vi "Main_v1.vi"() -> ()   [LabVIEW 2018, in "Application.lvlib"]
doc: "This VI is the main application VI in the Delacor QMH project template. This application VI is implemented as a simple state machine, which communicates with two different Delacor QMH modules.\n_____\nBased on DQMH Project Template 6.0.0.91."
uses:
  Application.lvlib
  Application Data--cluster.ctl
  Switches Module/MB switches Module.lvlib
  CE14 eMIC module/CE14 eMIC module.lvlib
  App States.ctl
  MB 01 switches Module/MB 01 switches Module.lvlib
  DMM Module/DMM Module.lvlib
  CE14  Module/CE14  Module.lvlib
  DRV cluster.ctl
  type defs/HW config.ctl
  Instrument Drivers/LVdriver_CE14(eMIC)/type defs/CE14.data.ctl
  Instrument Drivers/LVdriver_CE14(eMIC)/CE14_eMIC.lvlib
panel:
  out "eMIC response":T1[](array[typedef])
  out "time string":string
  out "Module ID":i32
  in  "Read ACI, ACV  from  eMIC(x6)":bool
  out "DCI":dbl
  out "DCV":dbl
  in  "Sets to Display":u16(ring)=2 items=["1st Display", "2nd Display", "1st & 2nd Display"]
  in  "Read DCI, DCV  from DMM":bool
  in  "Detector Rate":u8(ring)=2 items=["SLOW", "MID", "FAST"]
  in  "DCI range":dbl=10.0
  in  "DCV range":dbl=1000.0
  in  "config DMM":bool
  in  "mux2-1(DMM I) encode":enum16{"DMM I (0.5)", "DMM I (12)"}(ring)
  in  "DMM input Selection":bool
  in  "mux6_1(3wires)_encode":T2(ring)
  in  "mux6-1(x1)":bool
  in  "Time duration(ms)":i32
  in  "mux10_1(x6)_encode":T3(ring)
  in  "mux10-1(x6)":bool
  in  "eMIC (x6)":bool[](array[boolean])=[FALSE, FALSE, FALSE, FALSE, FALSE, FALSE]
  in  "eMIC":bool
  in  "demux1_10(x6)":T4(ring)
  in  "demux1-10(x6)":bool
  in  "SC enable":bool=TRUE
  in  "SC Enable":bool
  in  "M054 Close":bool
  in  "Arduino Close":bool
  in  "DMM Close":bool
  in  "M054 name":refnum<visa-resource-name>="COM11"
  in  "Arduino name":refnum<visa-resource-name>="COM16"
  in  "DMM name":refnum<visa-resource-name>="COM15"
  in  "M054 connect":bool
  in  "Arduino connect":bool
  in  "DMM connect":bool
  in  "Test":bool caption="Again"
  out "DMM Module Running?":bool
  out "MB01 Module Running?":bool
  in  "Start DMM Module Module":bool
  in  "Start MB01 Module Module":bool
  out "DRV 61":u32(colorbox)
  in  "Exit":bool
  in  "Pause":bool
  in  "Again":bool
  out "DRV 60":u32(colorbox) caption="60"
  out "DRV 59":u32(colorbox) caption="59"
  out "DRV 58":u32(colorbox) caption="58"
  out "DRV 57":u32(colorbox) caption="57"
  out "DRV 56":u32(colorbox) caption="56"
  out "DRV 55":u32(colorbox) caption="55"
  out "DRV 54":u32(colorbox) caption="54"
  out "DRV 53":u32(colorbox) caption="53"
  out "DRV 52":u32(colorbox) caption="52"
  out "DRV 51":u32(colorbox) caption="51"
  out "DRV 50":u32(colorbox) caption="50"
  out "DRV 49":u32(colorbox) caption="49"
  out "DRV 48":u32(colorbox) caption="48"
  out "DRV 47":u32(colorbox) caption="47"
  out "DRV 46":u32(colorbox) caption="46"
  out "DRV 45":u32(colorbox) caption="45"
  out "DRV 44":u32(colorbox) caption="44"
  out "DRV 43":u32(colorbox) caption="43"
  out "DRV 42":u32(colorbox) caption="42"
  out "DRV 41":u32(colorbox) caption="41"
  out "DRV 40":u32(colorbox) caption="40"
  out "DRV 39":u32(colorbox) caption="39"
  out "DRV 38":u32(colorbox) caption="38"
  out "DRV 37":u32(colorbox) caption="37"
  out "DRV 36":u32(colorbox) caption="36"
  out "DRV 35":u32(colorbox) caption="35"
  out "DRV 34":u32(colorbox) caption="34"
  out "DRV 33":u32(colorbox) caption="33"
  out "DRV 32":u32(colorbox) caption="32"
  out "DRV 31":u32(colorbox) caption="31"
  out "DRV 30":u32(colorbox) caption="30"
  out "DRV 29":u32(colorbox) caption="29"
  out "DRV 28":u32(colorbox) caption="28"
  out "DRV 27":u32(colorbox) caption="27"
  out "DRV 26":u32(colorbox) caption="26"
  out "DRV 25":u32(colorbox) caption="25"
  out "DRV 24":u32(colorbox) caption="24"
  out "DRV 23":u32(colorbox) caption="23"
  out "DRV 22":u32(colorbox) caption="22"
  out "DRV 21":u32(colorbox) caption="21"
  out "DRV 20":u32(colorbox) caption="20"
  out "DRV 19":u32(colorbox)=4375612 caption="19"
  out "DRV 18":u32(colorbox) caption="18"
  out "DRV 17":u32(colorbox) caption="17"
  out "DRV 16":u32(colorbox) caption="16"
  out "DRV 15":u32(colorbox) caption="15"
  out "DRV 14":u32(colorbox) caption="14"
  out "DRV 13":u32(colorbox)=4375612 caption="13"
  out "DRV 12":u32(colorbox) caption="12"
  out "DRV 11":u32(colorbox) caption="11"
  out "DRV 10":u32(colorbox) caption="10"
  out "DRV 9":u32(colorbox) caption="9"
  out "DRV 8":u32(colorbox) caption="8"
  out "DRV 7":u32(colorbox)=4375612 caption="7"
  out "DRV 6":u32(colorbox) caption="6"
  out "DRV 5":u32(colorbox) caption="5"
  out "DRV 4":u32(colorbox) caption="4"
  out "DRV 3":u32(colorbox) caption="3"
  out "DRV 2":u32(colorbox) caption="2"
  out "DRV 1":u32(colorbox)=13224393 caption="1"
  out "version":string caption="Version"
  in  "Hide Switches Module Module":bool
  in  "Show Switches Module Module":bool
  in  "Hide CE14 eMIC module Module":bool
  in  "Show CE14 eMIC module Module":bool
  in  "Stop CE14 eMIC module Module":bool
  in  "Stop Switches Module Module":bool
  in  "Start Switches Module Module":bool
  out "Active CE14 eMIC module Modules":string[](array[string])
  in  "Start New Instance CE14 eMIC module Module":bool
  in  "Select CE14 eMIC module Module Instance":i32(ring)=-1 items=["All"=-1]
  in  "Switches Module Module: Do Something Else":dbl caption="Do Something Else"
  in  "Switches Module Module: Do Something":bool
  out "Switches Module Running?":bool
  out "Status":string
  # "HV-60D: LED POWER DRIVER ON-LINE TESTER"
  # "DCI range:  10mV; 100mV;  1A, 10A"
  # "DCV range: 100mV/1V; 10V, 1000V"
  # "This top-level application allows you to launch and control a singleton module, and multiple instances of a cloneable module."
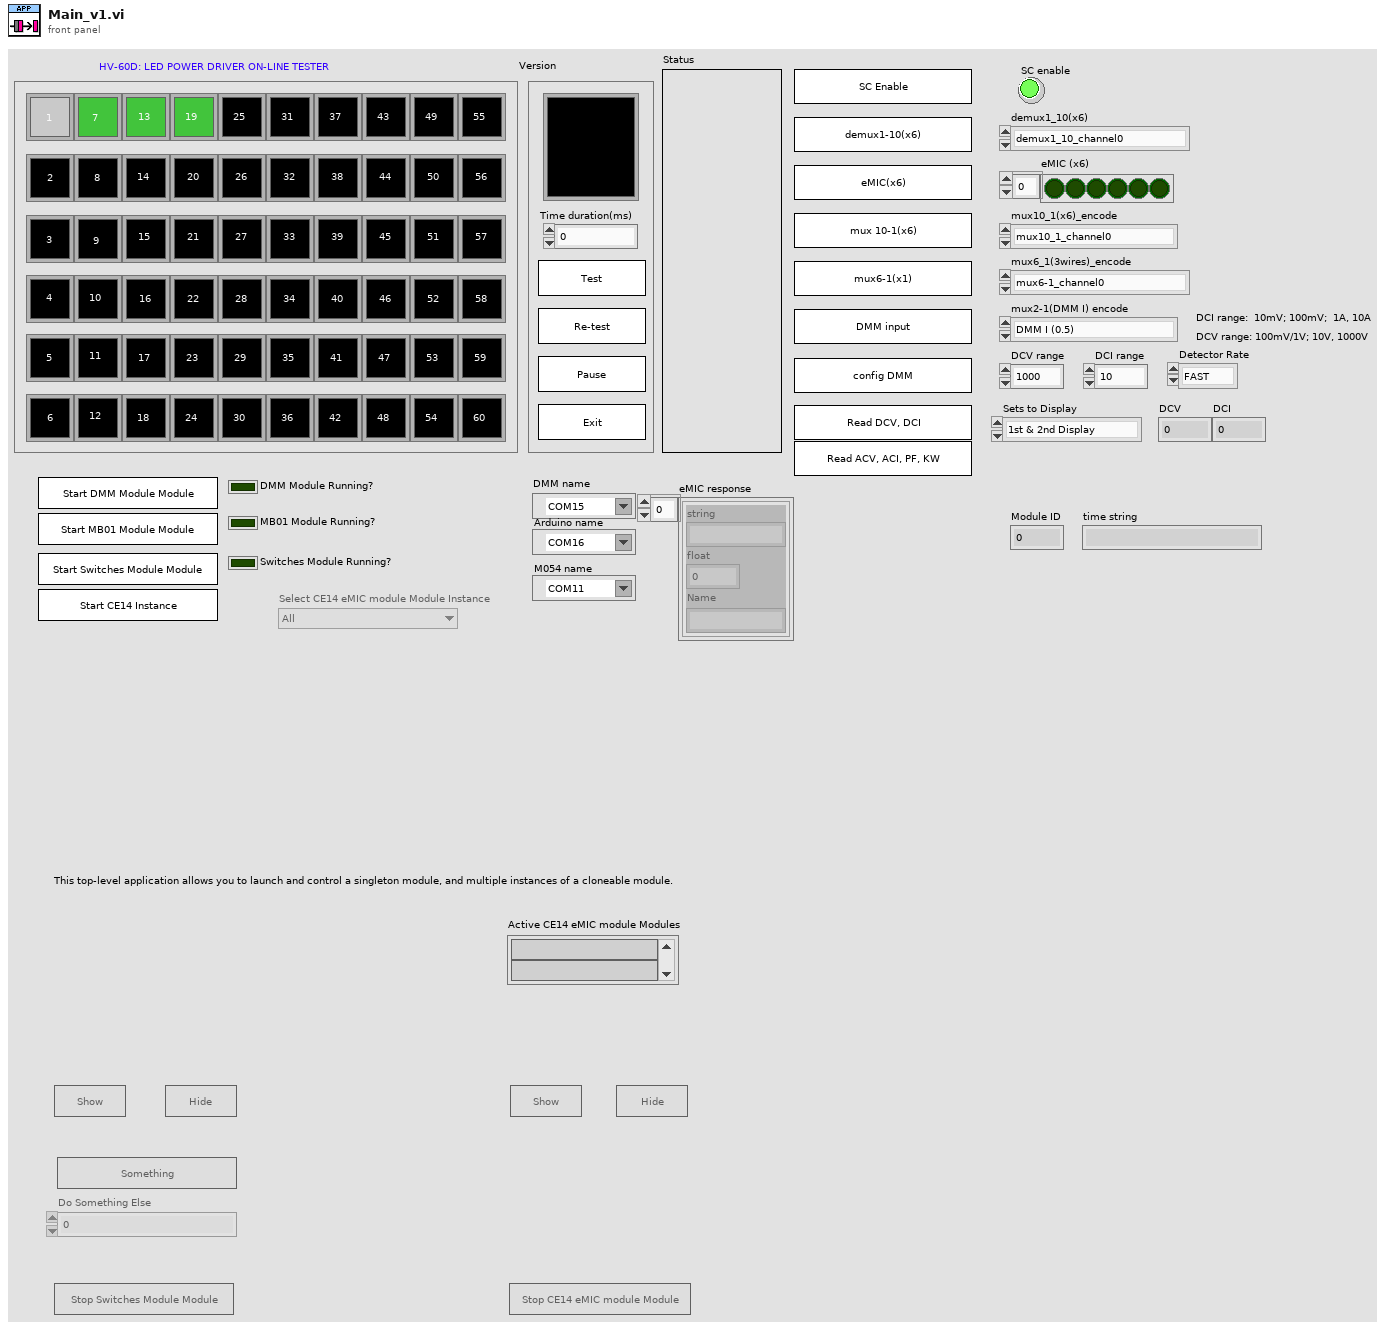
[diagram p1: front panel]
types:
  T1 = typedef "CE14_eMIC.lvlib/CE14.data.ctl" = cluster{"string":string, "float":dbl, "Name":string}
  T2 = enum16{"mux6-1_channel0", "mux6_1_channel1_0", "mux6_1_channel1_1", "mux6-1_channel1_2", "mux6_1_channel1_3", "mux6_1_channel2_0", "mux6_1_channel2_1", "mux6_1_channel2_2", "mux6_1_channel2_3", "mux6_1_channel3_0", "mux6_1_channel3_1", "mux6_1_channel3_2", "mux6_1_channel3_3", "mux6_1_channel4_0", "mux6_1_channel4_1", "mux6_1_channel4_2", "mux6_1_channel4_3", "mux6_1_channel5_0", "mux6_1_channel5_1", "mux6_1_channel5_2", "mux6_1_channel5_3", "mux6_1_channel6_0", "mux6_1_channel6_1", "mux6_1_channel6_2", "mux6_1_channel6_3"}
  T3 = enum16{"mux10_1_channel0", "mux10_1_channel1", "mux10_1_channel2", "mux10_1_channel3", "mux10_1_channel4", "mux10_1_channel5", "mux10_1_channel6", "mux10_1_channel7", "mux10_1_channel8", "mux10_1_channel9", "mux10_1_channel10"}
  T4 = enum16{"demux1_10_channel0", "demux1_10_channel1", "demux1_10_channel2", "demux1_10_channel3", "demux1_10_channel4", "demux1_10_channel5", "demux1_10_channel6", "demux1_10_channel7", "demux1_10_channel8", "demux1_10_channel9", "demux1_10_channel10"}
  T5 = typedef "Application.lvlib/App States.ctl" = enum16{"Apps.Initialize0", "Apps.Initialize1", "Apps.Initialize2", "Apps.Initialize3", "Apps.Initialize4", "Apps.Initialize Panel", "Apps.UI Interlocks", "Apps.UI.Reinitiatize", "Apps.Update Status", "Apps.Wait for Event", "Apps.Exit"}
  T6 = typedef "Application.lvlib/Application Data--cluster.ctl" = cluster{"Status":string, "Singleton Controls":refnum<vi>[], "Cloneable Controls":refnum<vi>[], "Module Ring Value":i32, "HW config":T7, "DUT values":T8[]}
  T7 = typedef "Application.lvlib/HW config.ctl" = cluster{"DMM":string, "mux":string, "demux":string, "eMIC1":string, "eMIC2":string, "eMIC3":string, "eMIC4":string, "eMIC5":string, "eMIC6":string}
  T8 = typedef "Application.lvlib/DRV cluster.ctl" = cluster{"Pass/Fail?":bool, "AC Characteristic":cluster{"Pass/Fail?":bool, "Voltage":cluster{"pass/fail?":bool, "Measured Value":dbl, "Upper Level":dbl, "Lower Level":dbl}, "Current":cluster{"pass/fail?":bool, "Measured Value":dbl, "Upper Level":dbl, "Lower Level":dbl}, "Power factor":cluster{"pass/fail?":bool, "Measured Value":dbl, "Upper Level":dbl, "Lower Level":dbl}, "Shorted Circuit":cluster{"Pass/Fail?":bool}}, "DC Characteristic":cluster{"Pass/Fail?":bool, "Voltage":cluster{"pass/fail?":bool, "Measured Value":dbl, "Upper Level":dbl, "Lower Level":dbl}, "Current":cluster{"pass/fail?":bool, "Measured Value":dbl, "Upper Level":dbl, "Lower Level":dbl}}}
  T9 = typedef "CE14  Module.lvlib/Broadcast Events--cluster.ctl" = cluster{"Module Did Init":refnum<user-event>, "Status Updated":refnum<user-event>, "Error Reported":refnum<user-event>, "Module Did Stop":refnum<user-event>, "Update Module Execution Status":refnum<user-event>, "eMICs response":refnum<user-event>}
  T10 = typedef "MB switches Module.lvlib/Broadcast Events--cluster.ctl" = cluster{"Module Did Init":refnum<user-event>, "Status Updated":refnum<user-event>, "Error Reported":refnum<user-event>, "Module Did Stop":refnum<user-event>, "Update Module Execution Status":refnum<user-event>}
  T11 = typedef "MB 01 switches Module.lvlib/Broadcast Events--cluster.ctl" = cluster{"Module Did Init":refnum<user-event>, "Status Updated":refnum<user-event>, "Error Reported":refnum<user-event>, "Module Did Stop":refnum<user-event>, "Update Module Execution Status":refnum<user-event>}
  T12 = typedef "DMM Module.lvlib/Broadcast Events--cluster.ctl" = cluster{"Module Did Init":refnum<user-event>, "Status Updated":refnum<user-event>, "Error Reported":refnum<user-event>, "Module Did Stop":refnum<user-event>, "Update Module Execution Status":refnum<user-event>}
  T13 = typedef "Application.lvlib/App States.ctl" = enum16{"Initialize", "Initialize Panel", "UI Interlocks", "Update Status", "Wait for Event", "Exit"}
  T14 = enum8{"Enabled", "Disabled", "Disabled and Grayed Out"}
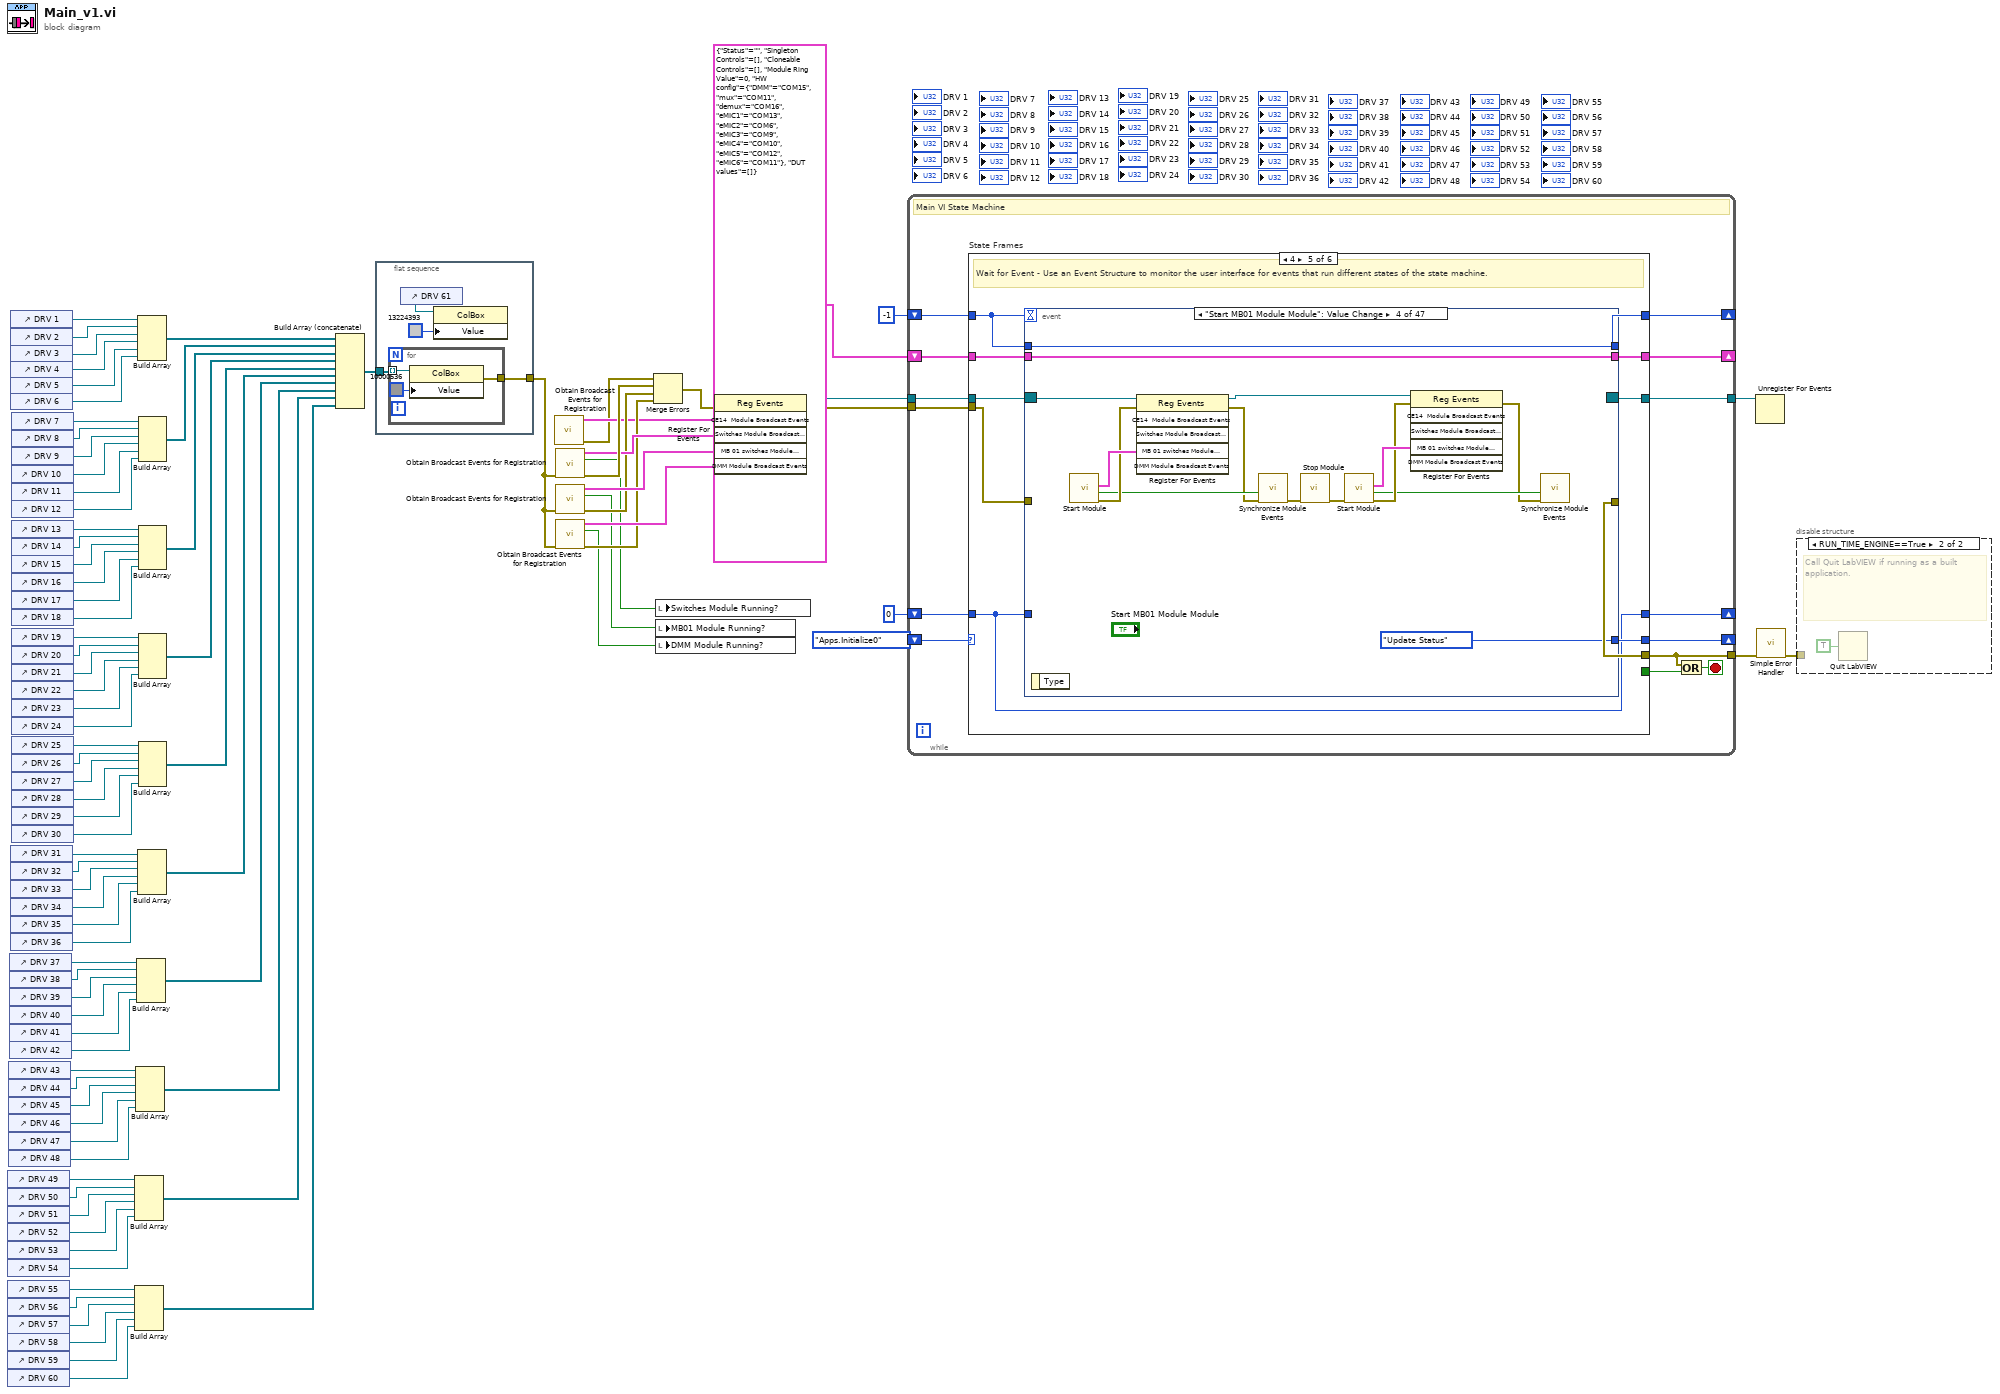
[diagram p0: block diagram]
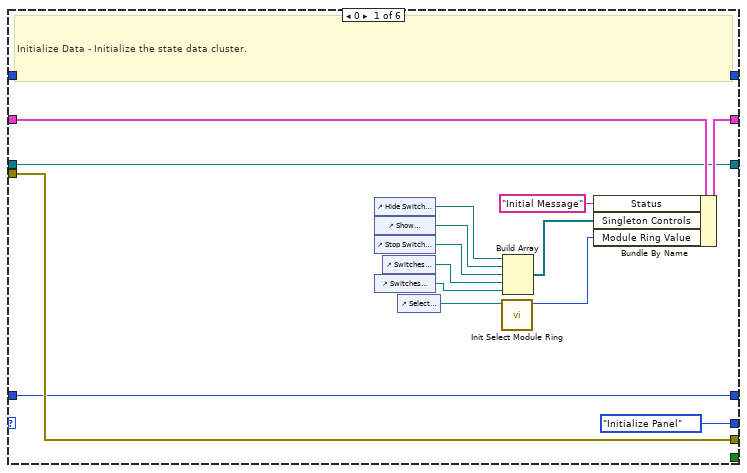
[diagram p2: hidden frame]
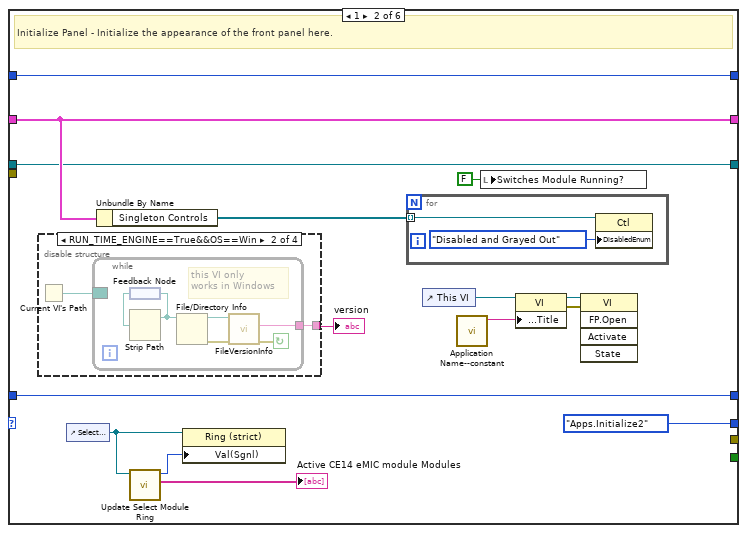
[diagram p3: hidden frame]
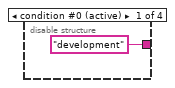
[diagram p4: hidden frame]
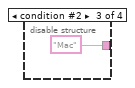
[diagram p5: hidden frame]
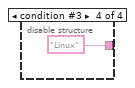
[diagram p6: hidden frame]
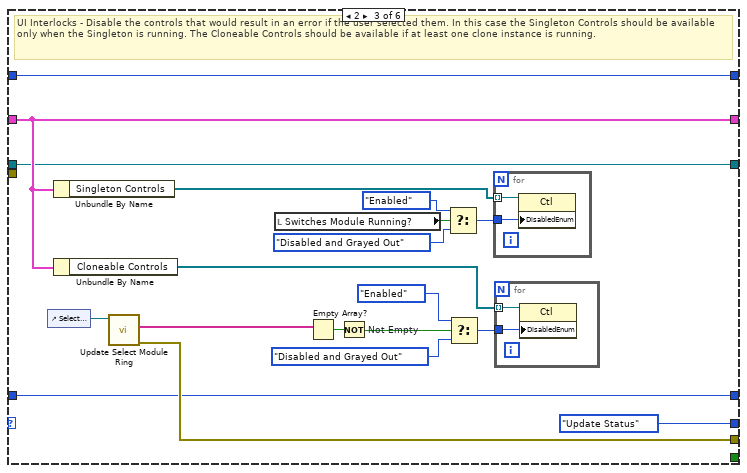
[diagram p7: hidden frame]
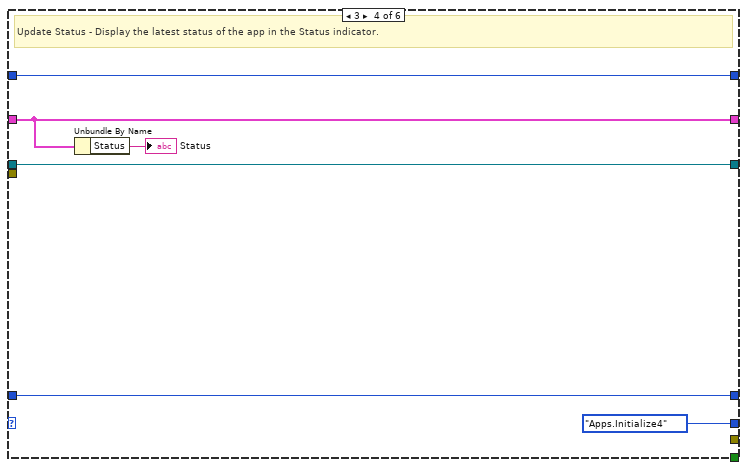
[diagram p8: hidden frame]
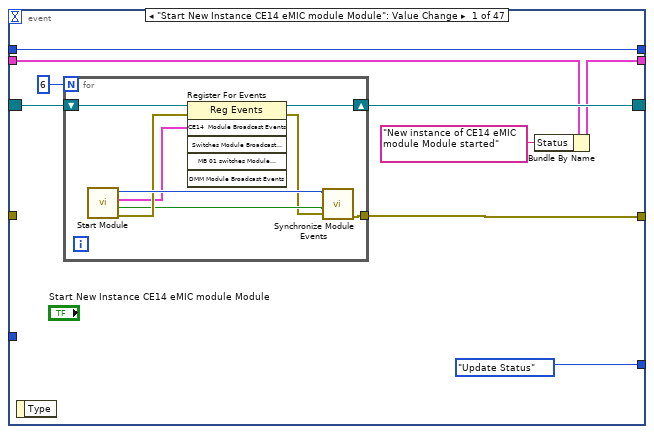
[diagram p9: hidden frame]
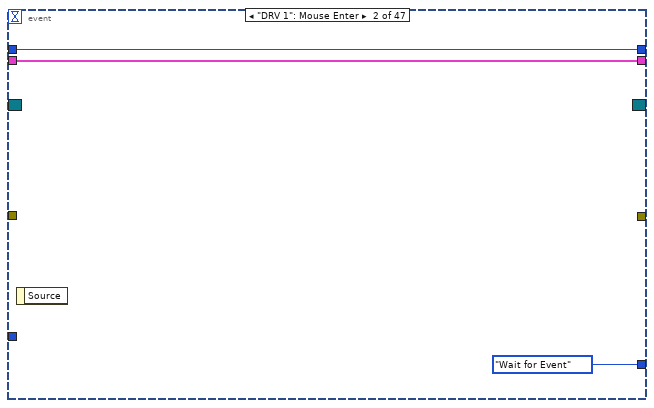
[diagram p10: hidden frame]
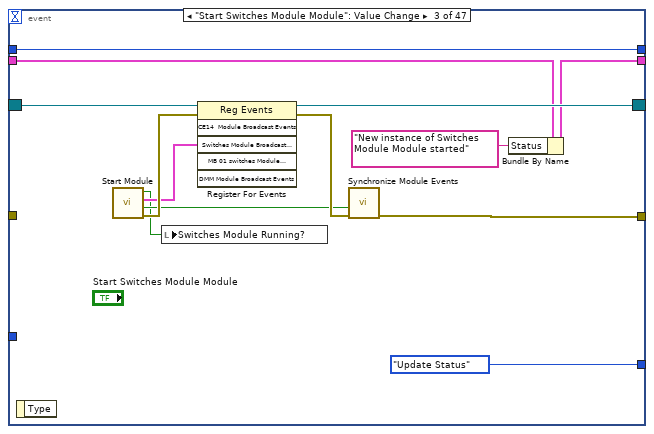
[diagram p11: hidden frame]
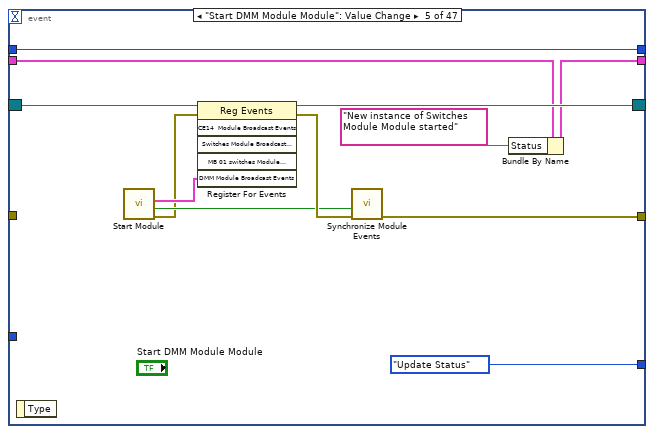
[diagram p12: hidden frame]
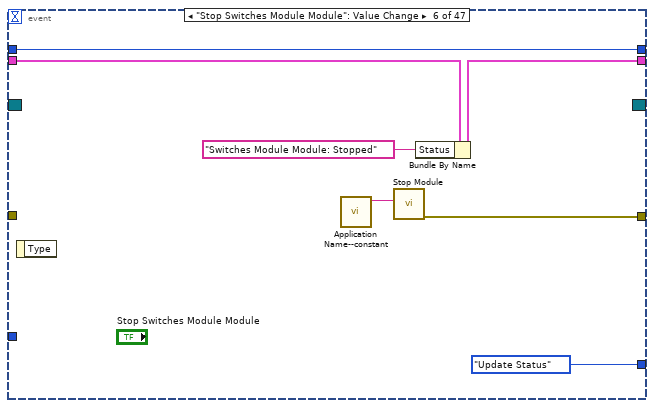
[diagram p13: hidden frame]
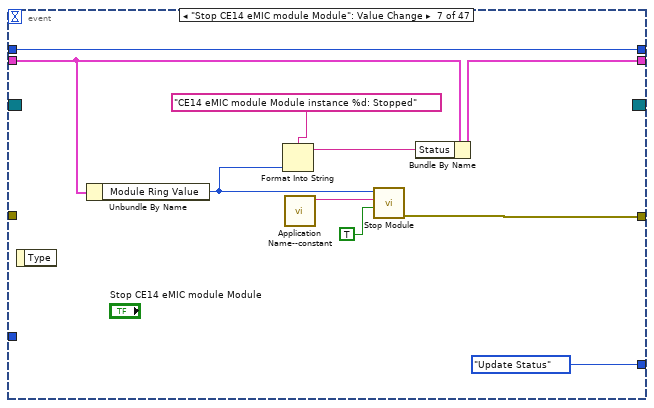
[diagram p14: hidden frame]
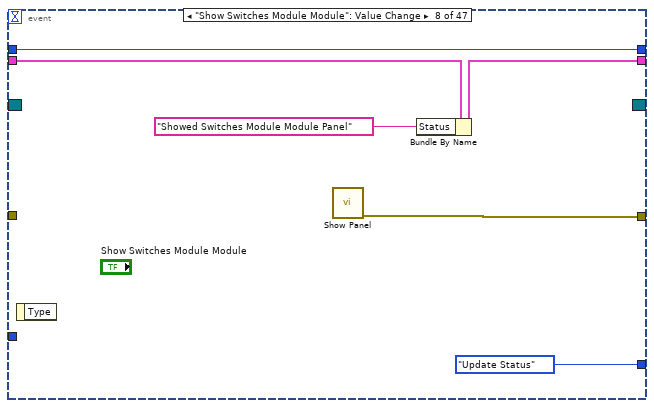
[diagram p15: hidden frame]
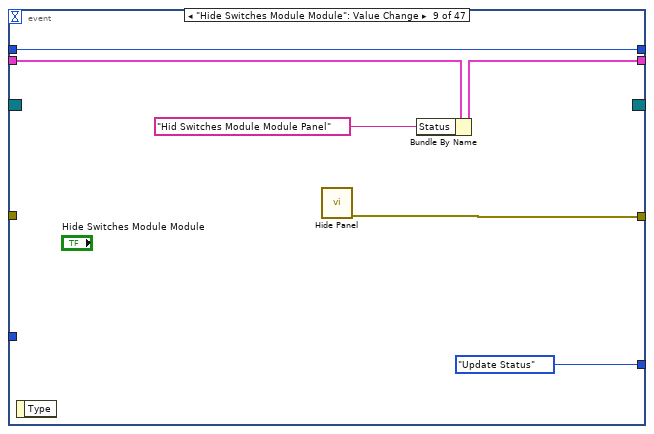
[diagram p16: hidden frame]
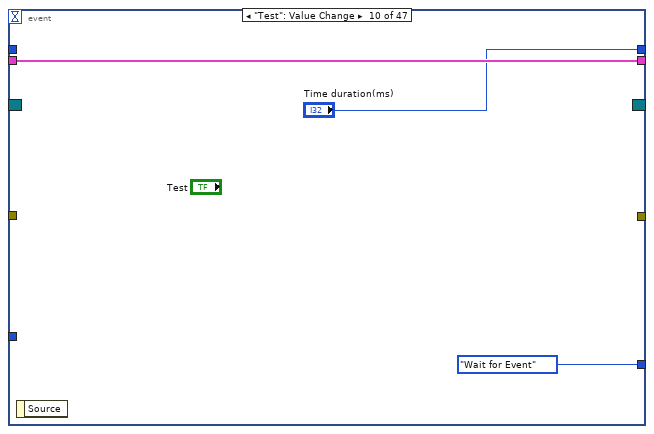
[diagram p17: hidden frame]
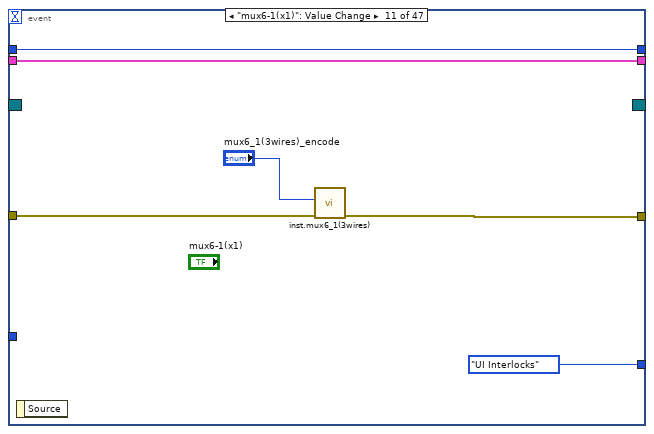
[diagram p18: hidden frame]
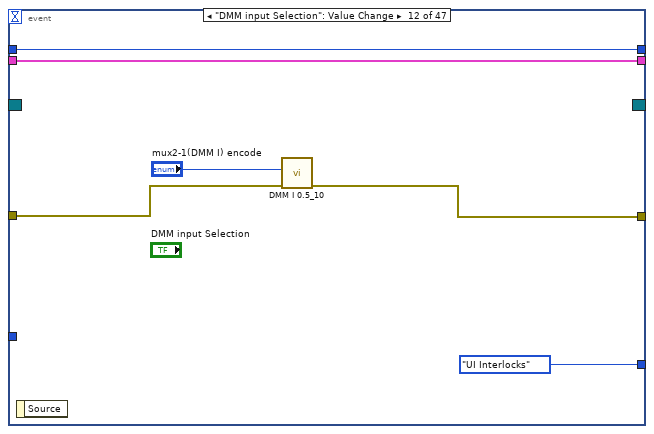
[diagram p19: hidden frame]
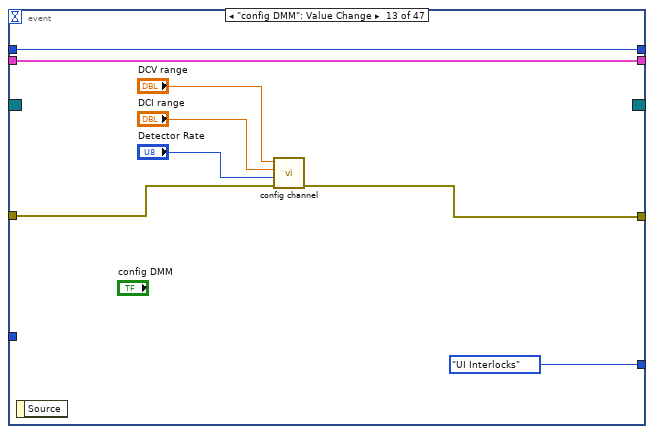
[diagram p20: hidden frame]
diagram:
  n1 = control-ref of="DRV 49"() -> (w25:refnum<vi>)
  n2 = control-ref of="DRV 50"() -> (w26:refnum<vi>)
  n3 = control-ref of="DRV 51"() -> (w27:refnum<vi>)
  n4 = control-ref of="DRV 52"() -> (w28:refnum<vi>)
  n5 = control-ref of="DRV 53"() -> (w29:refnum<vi>)
  n6 = control-ref of="DRV 54"() -> (w30:refnum<vi>)
  n7 = control-ref of="DRV 55"() -> (w24:refnum<vi>)
  n8 = control-ref of="DRV 56"() -> (w23:refnum<vi>)
  n9 = control-ref of="DRV 57"() -> (w22:refnum<vi>)
  n10 = control-ref of="DRV 58"() -> (w21:refnum<vi>)
  n11 = control-ref of="DRV 59"() -> (w20:refnum<vi>)
  n12 = control-ref of="DRV 60"() -> (w19:refnum<vi>)
  n13 = control-ref of="DRV 43"() -> (w36:refnum<vi>)
  n14 = control-ref of="DRV 44"() -> (w35:refnum<vi>)
  n15 = control-ref of="DRV 45"() -> (w34:refnum<vi>)
  n16 = control-ref of="DRV 46"() -> (w33:refnum<vi>)
  n17 = control-ref of="DRV 47"() -> (w32:refnum<vi>)
  n18 = control-ref of="DRV 48"() -> (w31:refnum<vi>)
  n19 = control-ref of="DRV 37"() -> (w37:refnum<vi>)
  n20 = control-ref of="DRV 38"() -> (w38:refnum<vi>)
  n21 = control-ref of="DRV 39"() -> (w39:refnum<vi>)
  n22 = control-ref of="DRV 40"() -> (w40:refnum<vi>)
  n23 = control-ref of="DRV 41"() -> (w41:refnum<vi>)
  n24 = control-ref of="DRV 42"() -> (w42:refnum<vi>)
  n25 = control-ref of="DRV 1"() -> (w83:refnum<vi>)
  n26 = control-ref of="DRV 2"() -> (w82:refnum<vi>)
  n27 = control-ref of="DRV 3"() -> (w81:refnum<vi>)
  n28 = control-ref of="DRV 4"() -> (w80:refnum<vi>)
  n29 = control-ref of="DRV 5"() -> (w79:refnum<vi>)
  n30 = control-ref of="DRV 6"() -> (w78:refnum<vi>)
  n31 = control-ref of="DRV 31"() -> (w48:refnum<vi>)
  n32 = control-ref of="DRV 32"() -> (w47:refnum<vi>)
  n33 = control-ref of="DRV 33"() -> (w46:refnum<vi>)
  n34 = control-ref of="DRV 34"() -> (w45:refnum<vi>)
  n35 = control-ref of="DRV 35"() -> (w44:refnum<vi>)
  n36 = control-ref of="DRV 36"() -> (w43:refnum<vi>)
  n37 = control-ref of="DRV 7"() -> (w72:refnum<vi>)
  n38 = control-ref of="DRV 8"() -> (w71:refnum<vi>)
  n39 = control-ref of="DRV 9"() -> (w70:refnum<vi>)
  n40 = control-ref of="DRV 10"() -> (w69:refnum<vi>)
  n41 = control-ref of="DRV 11"() -> (w68:refnum<vi>)
  n42 = control-ref of="DRV 12"() -> (w67:refnum<vi>)
  n43 = control-ref of="DRV 13"() -> (w61:refnum<vi>)
  n44 = control-ref of="DRV 14"() -> (w62:refnum<vi>)
  n45 = control-ref of="DRV 15"() -> (w63:refnum<vi>)
  n46 = control-ref of="DRV 16"() -> (w64:refnum<vi>)
  n47 = control-ref of="DRV 17"() -> (w65:refnum<vi>)
  n48 = control-ref of="DRV 18"() -> (w66:refnum<vi>)
  n49 = control-ref of="DRV 19"() -> (w60:refnum<vi>)
  n50 = control-ref of="DRV 20"() -> (w59:refnum<vi>)
  n51 = control-ref of="DRV 21"() -> (w58:refnum<vi>)
  n52 = control-ref of="DRV 22"() -> (w57:refnum<vi>)
  n53 = control-ref of="DRV 23"() -> (w56:refnum<vi>)
  n54 = control-ref of="DRV 24"() -> (w55:refnum<vi>)
  n55 = control-ref of="DRV 25"() -> (w49:refnum<vi>)
  n56 = control-ref of="DRV 26"() -> (w50:refnum<vi>)
  n57 = control-ref of="DRV 27"() -> (w51:refnum<vi>)
  n58 = control-ref of="DRV 28"() -> (w52:refnum<vi>)
  n59 = control-ref of="DRV 29"() -> (w53:refnum<vi>)
  n60 = control-ref of="DRV 30"() -> (w54:refnum<vi>)
  n61 = Build Array(w25, w26, w27, w28, w29, w30) -> (w10:refnum<vi>[])
  n62 = Build Array(w24, w23, w22, w21, w20, w19) -> (w9:refnum<vi>[])
  n63 = Build Array(w36, w35, w34, w33, w32, w31) -> (w11:refnum<vi>[])
  n64 = Build Array(w37, w38, w39, w40, w41, w42) -> (w12:refnum<vi>[])
  n65 = Build Array(w83, w82, w81, w80, w79, w78) -> (w18:refnum<vi>[])
  n66 = Build Array(w48, w47, w46, w45, w44, w43) -> (w13:refnum<vi>[])
  n67 = Build Array(w72, w71, w70, w69, w68, w67) -> (w17:refnum<vi>[])
  n68 = Build Array(w61, w62, w63, w64, w65, w66) -> (w16:refnum<vi>[])
  n69 = Build Array(w60, w59, w58, w57, w56, w55) -> (w15:refnum<vi>[])
  n70 = Build Array(w49, w50, w51, w52, w53, w54) -> (w14:refnum<vi>[])
  n71 = Build Array (concatenate)(w18, w17, w16, w15, w14, w13, w12, w11, w10, w9) -> (w8:refnum<vi>[])
  n72 = flat-sequence {
    tunnel: w8 -> [w97]
    tunnel: [w96] -> w7
    frame #0 {
      n73 = for {
        tunnel: w97 -> [w99] mode=indexing
        tunnel: [w98] -> w96
        n74 = property class="ColBox"(reference=w99, "Value"=u32 10000536 ("DRV 1")) -> (error out=w98:errorcluster)  [unwired: 1 in, 1 out]
      }
      n75 = control-ref of="DRV 61"() -> (w95:refnum<vi>)
      n76 = property class="ColBox"(reference=w95, "Value"=u32 13224393 ("DRV 1")) -> ()  [unwired: 1 in, 2 out]
    }
  }
  n77 = call "Obtain Broadcast Events for Registration.vi"() -> ("error out"=w1:errorcluster, "CE14  Module Broadcast Events"=w2:T9)  [unwired: 9 in, 1 out]
  n78 = call "Obtain Broadcast Events for Registration.vi"("error in (no error)"=w7) -> ("error out"=w90:errorcluster, "Already running?"=w3:bool, "Switches Module Broadcast Events"=w88:T10)  [unwired: 8 in]
  n79 = call "Obtain Broadcast Events for Registration.vi"("error in (no error)"=w7) -> ("error out"=w76:errorcluster, "Already running?"=w4:bool, "MB 01 switches Module Broadcast Events"=w77:T11)  [unwired: 8 in]
  n80 = call "Obtain Broadcast Events for Registration.vi"("error in (no error)"=w7) -> ("error out"=w74:errorcluster, "Already running?"=w5:bool, "DMM Module Broadcast Events"=w75:T12)  [unwired: 8 in]
  n81 = Merge Errors(w1, w90, w76, w74) -> (w91:errorcluster)
  n82 = local write "Switches Module Running?"(w3) -> ()
  n83 = local write "MB01 Module Running?"(w4) -> ()
  n84 = local write "DMM Module Running?"(w5) -> ()
  n85 = register-events(error in=w91, w2, w88, w77, w75) -> (reference out=w85:refnum<event-registration>, error out=w84:errorcluster)  [unwired: 1 in]
  n86 = while {
    shift-right: [w111] -> _
    shift-left: T6 {"Status"="", "Singleton Controls"=[], "Cloneable Controls"=[], "Module Ring Value"=0, "HW config"={"DMM"="COM15", "mux"="COM11", "demux"="COM16", "eMIC1"="COM13", "eMIC2"="COM6", "eMIC3"="COM9", "eMIC4"="COM10", "eMIC5"="COM12", "eMIC6"="COM11"}, "DUT values"=[]} ("Data Cluster") -> [w112]
    tunnel: [w114] -> w93
    shift-right: [w107] -> _
    shift-left: App_States."Apps.Initialize0" ("Initial State") -> [w109]
    tunnel: w84 -> [w113]
    tunnel: w85 -> [w106]
    tunnel: [w105] -> w86
    shift-right: [w103] -> _
    shift-left: 0 -> [w104]
    shift-right: [w101] -> _
    shift-left: -1 -> [w102]
    stop <- w108 stop-if-true
    # "Main VI State Machine"
    n87 = case "State Frames" shown="4" w109 {
      tunnel: [w130 _ w177 _ w197 w535] -> w114
      tunnel: w112 -> [w129 w142 w165 w187 w194 w533]
      tunnel: [w128 w142 w165 w187 w193 w533] -> w111
      tunnel: [_ _ _ _ _ w532] -> w110
      tunnel: [App_States."Initialize Panel" ("State") App_States."Apps.Initialize2" ("State") App_States."Update Status" ("State") App_States."Apps.Initialize4" ("State") w192 App_States."Apps.Initialize Panel" ("State")] -> w107
      tunnel: w106 -> [w118 w139 w161 w184 w196 w530]
      tunnel: [w118 w139 w161 w184 w195 w530] -> w105
      tunnel: w113 -> [w130 _ _ _ w191 _]
      tunnel: w104 -> [w117 w133 w160 w183 w190 w527]
      tunnel: [w117 w133 w160 w183 w190 w527] -> w103
      tunnel: w102 -> [w116 w131 w159 w182 w189 w526]
      tunnel: [w116 w131 w159 w182 w188 w526] -> w101
      frame 0 {
        # "Initialize Data - Initialize the state data cluster."
        n88 = control-ref of="Hide Switches Module Module"() -> (w126:refnum<vi>)
        n89 = control-ref of="Show Switches Module Module"() -> (w125:refnum<vi>)
        n90 = control-ref of="Stop Switches Module Module"() -> (w124:refnum<vi>)
        n91 = control-ref of="Switches Module Module: Do Something"() -> (w122:refnum<vi>)
        n92 = control-ref of="Switches Module Module: Do Something Else"() -> (w123:refnum<vi>)
        n93 = control-ref of="Select CE14 eMIC module Module Instance"() -> (w119:refnum<vi>)
        n94 = call "Init Select Module Ring.vi"("Select Module Ring Ref"=w119) -> ("Value for All Modules"=w115:i32)  [unwired: 8 in, 2 out]
        n95 = Build Array(w126, w125, w124, w123, w122) -> (w121:refnum<vi>[])
        n96 = Bundle By Name(cluster=w129, "Status"="Initial Message" ("Initial Message"), "Singleton Controls"=w121, "Module Ring Value"=w115) -> (w128:T6)
      }
      frame 1 {
        # "Initialize Panel - Initialize the appearance of the front panel here."
        n97 = disable-structure "Conditional Disable Structure" shown="RUN_TIME_ENGINE==True&&OS==Win" {
          disable-tunnel: ["development" w147 "Mac" "Linux"] -> w136
          frame condition #0 (active) {
          }
          frame condition #1 {
            n98 = Current VI's Path() -> (path=w148:path)
            n99 = while {
              border: w148 -> [_]
              tunnel: [w149] -> w147
              stop <- w153 continue-if-true
              # "this VI only \nworks in Windows"
              n100 = feedback #1() -> (w152:path)
              n101 = Strip Path(path=w152) -> (stripped path=w151:path)  [unwired: 1 out]
              n102 = feedback-in #1(w151) -> ()
              n103 = File/Directory Info(path=w151) -> (path out=w150:path, error out=w154:errorcluster)  [unwired: 1 in, 5 out]
              n104 = call <vilib>:"FileVersionInfo.vi"("error in (no error)"=w154, "Application Path in"=w150) -> ("error out"=w153:errorcluster, "File Version Info"=w149:string)  [unwired: 6 in, 2 out]
            }
          }
          frame condition #2 {
          }
          frame condition #3 {
          }
        }
        "version" <- w136
        n105 = control-ref of="Select CE14 eMIC module Module Instance"() -> (w138:refnum<vi>)
        n106 = Unbundle By Name(w142) -> ("Singleton Controls"=w141:refnum<vi>[])
        n107 = call "Update Select Module Ring.vi"("Select Module Ring Ref"=w138) -> ("Active Modules (Array)"=→"Active CE14 eMIC module Modules":string[], "New Module Ring Value"=w137:i32)  [unwired: 8 in, 1 out]
        n108 = property on="Property Node" class="Ring (strict)"(reference=w138, "Val(Sgnl)"=w137) -> ()  [unwired: 1 in, 2 out]
        n109 = for {
          tunnel: w141 -> [w158] mode=indexing
          n110 = property on="Property Node" class="Ctl"(reference=w158, "DisabledEnum"=T14."Disabled and Grayed Out" ("Disabled")) -> ()  [unwired: 1 in, 2 out]
        }
        n111 = control-ref of="This VI"() -> (w132:refnum<vi>)
        n112 = call "Application Name--constant.vi"() -> ("Application Name"=w135:string)  [unwired: 11 in]
        n113 = local write "Switches Module Running?"(FALSE ("My Singleton Module Init?")) -> ()
        n114 = property on="Property Node" class="VI"(reference=w132, "Front Panel.Title"=w135) -> (reference out=w134:refnum<vi>, error out=w145:errorcluster)  [unwired: 1 in]
        n115 = invoke class="VI" method="FP.Open"(reference=w134, error in=w145) -> ()  [unwired: 3 in, 5 out]
      }
      frame 2 {
        # "UI Interlocks - Disable the controls that would result in an error if the user selected them. In this case the Singleton Controls should be available only when the Singleton is running. The Cloneable Controls should be available if at least one clone instance is running."
        n116 = control-ref of="Select CE14 eMIC module Module Instance"() -> (w176:refnum<vi>)
        n117 = Unbundle By Name(w165) -> ("Singleton Controls"=w170:refnum<vi>[])
        n118 = Unbundle By Name(w165) -> ("Cloneable Controls"=w164:refnum<vi>[])
        n119 = call "Update Select Module Ring.vi"("Select Module Ring Ref"=w176) -> ("error out"=w177:errorcluster, "Active Modules (Array)"=w175:string[])  [unwired: 8 in, 1 out]
        n120 = local read "Switches Module Running?"() -> (w169:bool)
        n121 = Empty Array?(array=w175) -> (empty?=w174:bool)
        n122 = Not "Not Empty"(x=w174) -> (.not. x?=w163:bool)
        n123 = Select(t=T14."Enabled" ("Disabled"), s=w169, f=T14."Disabled and Grayed Out" ("Disabled")) -> (s? t:f=w171:T14)
        n124 = Select(t=T14."Enabled" ("Disabled"), s=w163, f=T14."Disabled and Grayed Out" ("Disabled")) -> (s? t:f=w168:T14)
        n125 = for {
          tunnel: w170 -> [w181] mode=indexing
          tunnel: w171 -> [w180]
          n126 = property on="Property Node" class="Ctl"(reference=w181, "DisabledEnum"=w180) -> ()  [unwired: 1 in, 2 out]
        }
        n127 = for {
          tunnel: w164 -> [w179] mode=indexing
          tunnel: w168 -> [w178]
          n128 = property on="Property Node" class="Ctl"(reference=w179, "DisabledEnum"=w178) -> ()  [unwired: 1 in, 2 out]
        }
      }
      frame 3 {
        # "Update Status - Display the latest status of the app in the Status indicator."
        n129 = Unbundle By Name(w187) -> ("Status"=→"Status":string)
      }
      frame 4 {
        # "Wait for Event - Use an Event Structure to monitor the user interface for events that run different states of the state machine."
        n130 = event shown="[3] \"Start MB01 Module Module\": Value Change" {
          selector: w196 -> [w206 _ w226 w245 w257 _ _ _ _ _ _ _ _ _ _ _ _ _ _ _ _ _ _ _ _ _ _ _ _ _ _ _ _ _ _ _ _ _ _ _ _ _ _ _ _ _ _]
          dyn-events: [w205 _ w225 _ w256 _ _ _ _ _ _ _ _ _ _ _ _ _ _ _ _ _ _ _ _ _ _ _ _ _ _ _ _ _ _ _ _ _ _ _ _ _ _ _ _ _ _] -> w195
          timeout: w189 -> [_ _ _ _ _ _ _ _ _ _ _ _ _ _ _ _ _ _ _ _ _ _ _ _ _ _ _ _ _ _ _ _ _ _ _ _ _ _ _ _ _ _ _ _ _ _ _]
          tunnel: [w199 _ w230 _ w247 w264 w266 w280 w286 _ w292 w298 w306 w314 w319 _ _ _ w335 w343 _ _ _ w369 w375 w380 w384 w388 w393 w400 w405 w412 w418 w424 w435 w445 _ _ w463 _ _ _ _ w506 _ _ _] -> w197
          tunnel: [w202 w217 w222 w237 w253 w260 w273 w278 w284 w289 w295 w301 w309 w317 w321 w328 w331 w334 w342 w350 w353 w359 w364 w371 w377 w382 w387 w391 w396 w402 w408 w414 w420 w426 w432 w442 w451 w458 w462 w466 w472 w483 w494 w499 w511 w517 w521] -> w193
          tunnel: w194 -> [w203 w217 w223 w237 w254 w261 w272 w279 w285 w289 w295 w301 w309 w317 w321 w328 w331 w334 w340 w348 w354 w360 w365 w371 w377 w382 w387 w391 w396 w402 w408 w414 w420 w426 w432 w442 w451 w458 w462 w467 w473 w484 w495 w502 w512 w517 w521]
          tunnel: [App_States."Update Status" ("State") App_States."Wait for Event" ("State") App_States."Update Status" ("State") App_States."Update Status" ("State") App_States."Update Status" ("State") App_States."Update Status" ("State") App_States."Update Status" ("State") App_States."Update Status" ("State") App_States."Update Status" ("State") App_States."Wait for Event" ("State") App_States."UI Interlocks" ("State") App_States."UI Interlocks" ("State") App_States."UI Interlocks" ("State") App_States."UI Interlocks" ("State") App_States."UI Interlocks" ("State") App_States."Wait for Event" ("State") App_States."Update Status" ("State") App_States."Wait for Event" ("State") App_States."Update Status" ("State") App_States."Update Status" ("State") App_States."Wait for Event" ("State") App_States."Wait for Event" ("State") App_States."Update Status" ("State") App_States."UI Interlocks" ("State") App_States."UI Interlocks" ("State") App_States."UI Interlocks" ("State") App_States."UI Interlocks" ("State") App_States."Wait for Event" ("State") App_States."UI Interlocks" ("State") App_States."UI Interlocks" ("State") App_States."UI Interlocks" ("State") App_States."UI Interlocks" ("State") App_States."UI Interlocks" ("State") App_States."UI Interlocks" ("State") App_States."UI Interlocks" ("State") App_States."UI Interlocks" ("State") App_States."UI Interlocks" ("State") App_States."UI Interlocks" ("State") App_States."UI Interlocks" ("State") App_States."Update Status" ("State") App_States."Update Status" ("State") App_States."Update Status" ("State") App_States."Update Status" ("State") App_States."UI Interlocks" ("State") App_States."UI Interlocks" ("State") App_States."Exit" ("State") App_States."Exit" ("State")] -> w192
          tunnel: w191 -> [_ _ _ _ _ _ _ _ _ _ w293 w299 w307 w315 _ _ _ _ _ _ _ _ _ w370 w376 w381 w385 w388 w394 w401 w406 w413 w419 w425 _ _ _ _ _ _ _ _ _ _ _ _ _]
          tunnel: w190 -> [_ _ _ _ _ _ _ _ _ _ _ _ _ _ _ _ _ _ _ _ _ _ _ _ _ _ _ _ _ _ _ _ _ _ _ _ _ _ _ _ _ _ _ _ _ _ _]
          tunnel: w189 -> [w200 w216 w218 w239 w246 w258 w269 w275 w281 _ w294 w300 w308 w316 w322 w327 _ _ w337 w345 w351 w356 w361 w366 w372 w378 w383 w390 w392 w397 w403 w409 w415 w421 w430 w440 w447 w452 w459 w465 w470 w475 w486 w497 w507 w515 w519]
          tunnel: [w200 w216 w218 w239 w246 w258 w269 w275 w281 "Time duration(ms)" w294 w300 w308 w316 w322 w327 -1 w333 w337 w345 w351 w356 w361 w366 w372 w378 w383 w390 w392 w397 w403 w409 w415 w421 w430 w440 w447 w452 w459 w465 w470 w475 w486 w497 w507 w515 w519] -> w188
          event "Start New Instance CE14 eMIC module Module": Value Change {
            n131 = event-data() -> ()  [unwired: 1 in, 1 out]
            n132 = for {
              N: 6 -> [_]
              tunnel: [w207] -> w199
              shift-right: [w213] -> w205
              shift-left: w206 -> [w214]
              n133 = call "Start Module.vi"() -> ("error out"=w211:errorcluster, "Wait for Event Sync?"=w209:bool, "CE14  Module Broadcast Events"=w210:T9, "Module ID"=w212:i32)  [unwired: 8 in]
              n134 = register-events(reference=w214, error in=w211, w210) -> (reference out=w213:refnum<event-registration>, error out=w208:errorcluster)  [unwired: 3 in]
              n135 = call "Synchronize Module Events.vi"("error in"=w208, "Wait for Event Sync?"=w209, "Module ID in"=w212) -> ("error out"=w207:errorcluster)  [unwired: 7 in, 1 out]
            }
            n136 = Bundle By Name(cluster=w203, "Status"="New instance of CE14 eMIC module Module started") -> (w202:T6)
          }
          event "DRV 1": Mouse Enter {
            n137 = event-data() -> ()  [unwired: 1 in, 1 out]
          }
          event "Start Switches Module Module": Value Change {
            n138 = event-data() -> ()  [unwired: 1 in, 1 out]
            n139 = call "Start Module.vi"() -> ("error out"=w229:errorcluster, "Wait for Event Sync?"=w227:bool, "Switches Module Broadcast Events"=w220:T10, "Module Was Already Running?"=w219:bool)  [unwired: 8 in]
            n140 = local write "Switches Module Running?"(w219) -> ()
            n141 = register-events(reference=w226, error in=w229, w220) -> (reference out=w225:refnum<event-registration>, error out=w228:errorcluster)  [unwired: 3 in]
            n142 = call "Synchronize Module Events.vi"("error in"=w228, "Wait for Event Sync?"=w227) -> ("error out"=w230:errorcluster)  [unwired: 9 in]
            n143 = Bundle By Name(cluster=w223, "Status"="New instance of Switches Module Module started") -> (w222:T6)
          }
          event "Start MB01 Module Module": Value Change {
            n144 = event-data() -> ()  [unwired: 1 in, 1 out]
            n145 = call "Start Module.vi"() -> ("error out"=w242:errorcluster, "Wait for Event Sync?"=w241:bool, "MB 01 switches Module Broadcast Events"=w243:T11)  [unwired: 8 in, 1 out]
            n146 = register-events(reference=w245, error in=w242, w243) -> (reference out=w232:refnum<event-registration>, error out=w240:errorcluster)  [unwired: 3 in]
            n147 = call "Synchronize Module Events.vi"("error in"=w240, "Wait for Event Sync?"=w241) -> ("error out"=w238:errorcluster)  [unwired: 9 in]
            n148 = call "Stop Module.vi"("error in"=w238) -> ("error out"=w231:errorcluster)  [unwired: 10 in]
            n149 = call "Start Module.vi"("error in (no error)"=w231) -> ("error out"=w235:errorcluster, "Wait for Event Sync?"=w234:bool, "MB 01 switches Module Broadcast Events"=w236:T11)  [unwired: 7 in, 1 out]
            n150 = register-events(reference=w232, error in=w235, w236) -> (error out=w233:errorcluster)  [unwired: 3 in, 1 out]
            n151 = call "Synchronize Module Events.vi"("error in"=w233, "Wait for Event Sync?"=w234) -> ()  [unwired: 9 in, 1 out]
          }
          event "Start DMM Module Module": Value Change {
            n152 = event-data() -> ()  [unwired: 1 in, 1 out]
            n153 = call "Start Module.vi"() -> ("error out"=w248:errorcluster, "Wait for Event Sync?"=w250:bool, "DMM Module Broadcast Events"=w249:T12)  [unwired: 8 in, 1 out]
            n154 = register-events(reference=w257, error in=w248, w249) -> (reference out=w256:refnum<event-registration>, error out=w251:errorcluster)  [unwired: 3 in]
            n155 = call "Synchronize Module Events.vi"("error in"=w251, "Wait for Event Sync?"=w250) -> ("error out"=w247:errorcluster)  [unwired: 9 in]
            n156 = Bundle By Name(cluster=w254, "Status"="New instance of Switches Module Module started") -> (w253:T6)
          }
          event "Stop Switches Module Module": Value Change {
            n157 = event-data() -> ()  [unwired: 1 in, 1 out]
            n158 = call "Application Name--constant.vi"() -> ("Application Name"=w262:string)  [unwired: 11 in]
            n159 = call "Stop Module.vi"("Origin"=w262) -> ("error out"=w264:errorcluster)  [unwired: 10 in]
            n160 = Bundle By Name(cluster=w261, "Status"="Switches Module Module: Stopped" ("Message")) -> (w260:T6)
          }
          event "Stop CE14 eMIC module Module": Value Change {
            n161 = event-data() -> ()  [unwired: 1 in, 1 out]
            n162 = Unbundle By Name(w272) -> ("Module Ring Value"=w268:i32)
            n163 = Format Into String(format string="CE14 eMIC module Module instance %d: Stopped" ("Message"), w268) -> (resulting string=w270:string)  [unwired: 2 in, 1 out]
            n164 = call "Application Name--constant.vi"() -> ("Application Name"=w267:string)  [unwired: 11 in]
            n165 = call "Stop Module.vi"("Wait for Module to stop? (F)"=TRUE, "Origin"=w267, "Module ID"=w268) -> ("error out"=w266:errorcluster)  [unwired: 8 in]
            n166 = Bundle By Name(cluster=w272, "Status"=w270) -> (w273:T6)
          }
          event "Show Switches Module Module": Value Change {
            n167 = event-data() -> ()  [unwired: 1 in, 1 out]
            n168 = call "Show Panel.vi"() -> ("error out"=w280:errorcluster)  [unwired: 11 in]
            n169 = Bundle By Name(cluster=w279, "Status"="Showed Switches Module Module Panel" ("Message")) -> (w278:T6)
          }
          event "Hide Switches Module Module": Value Change {
            n170 = event-data() -> ()  [unwired: 1 in, 1 out]
            n171 = call "Hide Panel.vi"() -> ("error out"=w286:errorcluster)  [unwired: 11 in]
            n172 = Bundle By Name(cluster=w285, "Status"="Hid Switches Module Module Panel" ("Message")) -> (w284:T6)
          }
          event "Test": Value Change {
            n173 = event-data() -> ()  [unwired: 1 in, 1 out]
          }
          event "mux6-1(x1)": Value Change {
            n174 = event-data() -> ()  [unwired: 1 in, 1 out]
            n175 = call "inst.mux6_1(3wires).vi"("error in"=w293, "mux6_1(3wires)_encode"="mux6_1(3wires)_encode") -> ("error out"=w292:errorcluster)  [unwired: 9 in]
          }
          event "DMM input Selection": Value Change {
            n176 = event-data() -> ()  [unwired: 1 in, 1 out]
            n177 = call "DMM I 0.5_10.vi"("error in"=w299, "mux2-1(DMM I) encode"="mux2-1(DMM I) encode") -> ("error out"=w298:errorcluster)  [unwired: 9 in]
          }
          event "config DMM": Value Change {
            n178 = event-data() -> ()  [unwired: 1 in, 1 out]
            n179 = call "config channel.vi"("error in"=w307, "Detector Rate"="Detector Rate", "DCI range"="DCI range", "DCV range"="DCV range") -> ("error out"=w306:errorcluster)  [unwired: 7 in]
          }
          event "Read DCI, DCV  from DMM": Value Change {
            n180 = event-data() -> ()  [unwired: 1 in, 1 out]
            n181 = call "Read DCV_DCI.vi"("error in"=w315, "Sets to Display"="Sets to Display") -> ("error out"=w314:errorcluster, "DCI"=→"DCI":dbl, "DCV"=→"DCV":dbl)  [unwired: 6 in, 1 out]
          }
          event "Read ACI, ACV  from  eMIC(x6)": Value Change {
            n182 = event-data() -> ()  [unwired: 1 in, 1 out]
            n183 = call "Read AC para.vi"("Module ID"=-1) -> ("error out"=w319:errorcluster)  [unwired: 10 in]
          }
          event User Event {
            n184 = event-data() -> ("Module ID"=→"Module ID":i32, "eMIC response"=→"eMIC response":T1[])  [unwired: 1 in]
            n185 = Get Date/Time String() -> (time string=→"time string":string)  [unwired: 3 in, 1 out]
          }
          event "Pause": Value Change {
            n186 = event-data() -> ()  [unwired: 1 in, 1 out]
          }
          event "Again": Value Change {
            n187 = event-data() -> ()  [unwired: 1 in, 1 out]
            n188 = local read "Time duration(ms)"() -> (w333:i32)
          }
          event "Show CE14 eMIC module Module": Value Change {
            n189 = event-data() -> ()  [unwired: 1 in, 1 out]
            n190 = Unbundle By Name(w340) -> ("Module Ring Value"=w336:i32)
            n191 = Format Into String(format string="CE14 eMIC module Module instance %d: Panel Shown" ("Message"), w336) -> (resulting string=w338:string)  [unwired: 2 in, 1 out]
            n192 = call "Show Panel.vi"("Module ID"=w336) -> ("error out"=w335:errorcluster)  [unwired: 10 in]
            n193 = Bundle By Name(cluster=w340, "Status"=w338) -> (w342:T6)
          }
          event "Hide CE14 eMIC module Module": Value Change {
            n194 = event-data() -> ()  [unwired: 1 in, 1 out]
            n195 = Unbundle By Name(w348) -> ("Module Ring Value"=w344:i32)
            n196 = call "Hide Panel.vi"("Module ID"=w344) -> ("error out"=w343:errorcluster)  [unwired: 10 in]
            n197 = Format Into String(format string="CE14 eMIC module Module instance %d: Panel Hidden" ("Message"), w344) -> (resulting string=w346:string)  [unwired: 2 in, 1 out]
            n198 = Bundle By Name(cluster=w348, "Status"=w346) -> (w350:T6)
          }
          event "Select CE14 eMIC module Module Instance": Value Change {
            # "Store new selected Module ID value in shift register."
            n199 = event-data() -> ()  [unwired: 1 in, 1 out]
            n200 = Bundle By Name(cluster=w354, "Module Ring Value"="Select CE14 eMIC module Module Instance") -> (w353:T6)
          }
          event "Switches Module Module: Do Something": Value Change {
            # "Send \"Do Something\" request to Switches Module Module"
            n201 = event-data() -> ()  [unwired: 1 in, 1 out]
            n202 = Bundle By Name(cluster=w360, "Status"="\"Something\" button pressed in top-level application VI" ("\"Do Something Else\" button pressed")) -> (w359:T6)
          }
          event "Switches Module Module: Do Something Else": Value Change {
            # "Send \"Do Something Else\" request to Switches Module Module"
            n203 = event-data() -> ()  [unwired: 1 in, 1 out]
            n204 = Bundle By Name(cluster=w365, "Status"="\"Do Something Else\" numeric value changed in top-level application VI. New value: " ("\"Do Something Else\" button pressed")) -> (w364:T6)
          }
          event "DMM connect": Value Change {
            n205 = event-data() -> ()  [unwired: 1 in, 1 out]
            n206 = call "DMM init.vi"("error in"=w370, "VISA resource name"="DMM name") -> ("error out"=w369:errorcluster)  [unwired: 9 in]
          }
          event "Arduino connect": Value Change {
            n207 = event-data() -> ()  [unwired: 1 in, 1 out]
            n208 = call "MB01 Open.vi"("error in"=w376, "VISA resource name"="Arduino name") -> ("error out"=w375:errorcluster)  [unwired: 9 in]
          }
          event "M054 Close": Value Change {
            n209 = event-data() -> ()  [unwired: 1 in, 1 out]
            n210 = call "inst.Close.vi"("error in"=w381) -> ("error out"=w380:errorcluster)  [unwired: 10 in]
          }
          event "DMM Close": Value Change {
            n211 = event-data() -> ()  [unwired: 1 in, 1 out]
            n212 = call "DMM Close.vi"("error in"=w385) -> ("error out"=w384:errorcluster)  [unwired: 10 in]
          }
          event Timeout {
            n213 = event-data() -> ()  [unwired: 1 in, 1 out]
          }
          event "Arduino Close": Value Change {
            n214 = event-data() -> ()  [unwired: 1 in, 1 out]
            n215 = call "MB01 Close.vi"("error in"=w394) -> ("error out"=w393:errorcluster)  [unwired: 10 in]
          }
          event "M054 connect": Value Change {
            n216 = event-data() -> ()  [unwired: 1 in, 1 out]
            n217 = call "inst.Open.vi"("error in"=w401, "VISA resource name"="M054 name") -> ("error out"=w400:errorcluster)  [unwired: 9 in]
          }
          event "SC Enable": Value Change {
            n218 = event-data() -> ()  [unwired: 1 in, 1 out]
            n219 = call "SC enable.vi"("error in"=w406, "5V enable"="SC enable") -> ("error out"=w405:errorcluster)  [unwired: 9 in]
          }
          event "demux1-10(x6)": Value Change {
            n220 = event-data() -> ()  [unwired: 1 in, 1 out]
            n221 = call "demux1-10.vi"("error in"=w413, "demux1_10(x6)_encode"="demux1_10(x6)") -> ("error out"=w412:errorcluster)  [unwired: 9 in]
          }
          event "eMIC": Value Change {
            n222 = event-data() -> ()  [unwired: 1 in, 1 out]
            n223 = call "MB01_eMICs.vi"("error in"=w419, "Array"="eMIC (x6)") -> ("error out"=w418:errorcluster)  [unwired: 9 in]
          }
          event "mux10-1(x6)": Value Change {
            n224 = event-data() -> ()  [unwired: 1 in, 1 out]
            n225 = call "inst.mux10_1.vi"("error in"=w425, "mux10_1(x6)_encode"="mux10_1(x6)_encode") -> ("error out"=w424:errorcluster)  [unwired: 9 in]
          }
          event User Event {
            # "A new instance of CE14 eMIC module Module has broadcast that is has been initialized"
            n226 = event-data() -> ("Info"=w434:string, "Module ID"=w431:i32)  [unwired: 1 in]
            n227 = control-ref of="Select CE14 eMIC module Module Instance"() -> (w429:refnum<vi>)
            n228 = local write "Status"(w434) -> ()
            n229 = call "Update Select Module Ring.vi"("Select Module Ring Ref"=w429) -> ("error out"=w427:errorcluster, "Active Modules (Array)"=w428:string[])  [unwired: 8 in, 1 out]
            n230 = local write "Active CE14 eMIC module Modules"(w428) -> ()
            n231 = disable-structure shown="Disabled" {
              disable-tunnel: [w438 w439] -> w435
              disable-tunnel: w427 -> [w437 w439]
              disable-tunnel: w431 -> [w436 _]
              frame Disabled {
                n232 = call "Show Panel.vi"("error in (no error)"=w437, "Module ID"=w436) -> ("error out"=w438:errorcluster)  [unwired: 9 in]
              }
              frame Enabled {
              }
            }
          }
          event User Event {
            # "Switches Module Module has broadcast that it has been initialized"
            n233 = event-data() -> ("Init?"=→"Switches Module Running?":bool, "Info"=w444:string)  [unwired: 1 in]
            n234 = local write "Status"(w444) -> ()
            n235 = disable-structure shown="Disabled" {
              disable-tunnel: [w446 _] -> w445
              frame Disabled {
                n236 = call "Show Panel.vi"() -> ("error out"=w446:errorcluster)  [unwired: 11 in]
              }
              frame Enabled {
              }
            }
          }
          event User Event {
            n237 = event-data() -> ("Init?"=→"DMM Module Running?":bool, "Info"=w449:string)  [unwired: 1 in]
            n238 = local write "Status"(w449) -> ()
          }
          event User Event {
            n239 = event-data() -> ("Init?"=→"MB01 Module Running?":bool, "Info"=w454:string)  [unwired: 1 in]
            n240 = Concatenate Strings(w454, "\r\n") -> (w453:string)
            n241 = local write "Status"(w453) -> ()
          }
          event User Event {
            # "Switches Module Module has broadcast its execution status"
            n242 = event-data() -> ("Running?"=w460:bool)  [unwired: 1 in]
            n243 = local write "Switches Module Running?"(w460) -> ()
            n244 = case shown="True" w460 {
              tunnel: [_ w464] -> w463
              frame False {
              }
              frame True {
                n245 = call "Show Panel.vi"() -> ("error out"=w464:errorcluster)  [unwired: 11 in]
              }
            }
          }
          event User Event {
            # "An instance of CE14 eMIC module Module has broadcast its status"
            n246 = event-data() -> ("Status"=w469:string)  [unwired: 1 in]
            n247 = Bundle By Name(cluster=w467, "Status"=w469) -> (w466:T6)
          }
          event User Event {
            # "Switches Module Module has broadcast its status"
            n248 = event-data() -> ("Status"=w474:string)  [unwired: 1 in]
            n249 = Bundle By Name(cluster=w473, "Status"=w474) -> (w472:T6)
          }
          event User Event {
            # "CE14 eMIC module Module had an error"
            n250 = event-data() -> ("Module Name"=w477:string, "Additional Information"=w480:string, "Error"=w485:errorcluster)  [unwired: 1 in]
            n251 = Unbundle By Name(w485) -> ("code"=w476:i32, "source"=w479:string)
            n252 = Format Into String(format string="Error code %d  Module: %s Additional Information: %s\nSource: %s", w476, w477, w480, w479) -> (resulting string=w478:string)  [unwired: 2 in, 1 out]
            n253 = Bundle By Name(cluster=w484, "Status"=w478) -> (w483:T6)
          }
          event User Event {
            # "Switches Module Module had an error"
            n254 = event-data() -> ("Module Name"=w488:string, "Additional Information"=w492:string, "Error"=w496:errorcluster)  [unwired: 1 in]
            n255 = Unbundle By Name(w496) -> ("code"=w487:i32, "source"=w491:string)
            n256 = Format Into String(format string="Error code %d Module: %s  Additional Information: %s\nSource: %s", w487, w488, w492, w491) -> (resulting string=w489:string)  [unwired: 2 in, 1 out]
            n257 = Bundle By Name(cluster=w495, "Status"=w489) -> (w494:T6)
          }
          event User Event {
            n258 = event-data() -> ("Origin"=w501:string)  [unwired: 1 in]
            n259 = Bundle By Name(cluster=w502, "Status"=w501) -> (w500:T6)
            n260 = control-ref of="Select CE14 eMIC module Module Instance"() -> (w505:refnum<vi>)
            n261 = call "Update Select Module Ring.vi"("Select Module Ring Ref"=w505) -> ("error out"=w506:errorcluster, "Active Modules (Array)"=w504:string[], "New Module Ring Value"=w498:i32)  [unwired: 8 in]
            n262 = Bundle By Name(cluster=w500, "Module Ring Value"=w498) -> (w499:T6)
            n263 = local write "Active CE14 eMIC module Modules"(w504) -> ()
          }
          event User Event {
            n264 = event-data() -> ("Origin"=w509:string)  [unwired: 1 in]
            n265 = local write "Switches Module Running?"(FALSE ("My Singleton Module Init?")) -> ()
            n266 = Concatenate Strings(w509, " Did Stop.") -> (w508:string)
            n267 = Bundle By Name(cluster=w512, "Status"=w508) -> (w511:T6)
          }
          event Panel Close? {
            # "Go to the 'Exit' state if the user tries to close the panel."
            n268 = event-data() -> ()  [unwired: 1 in, 1 out]
            n269 = event-data ("Event Filter Node")("Discard?"=TRUE) -> ()  [unwired: 1 in, 1 out]
          }
          event "Exit": Value Change {
            n270 = event-data() -> ()  [unwired: 1 in, 1 out]
          }
        }
      }
      frame 5 {
        w523 = TRUE  # Wait for Module to stop?
        w532 = TRUE  # Stop the VI
        # "Stop all modules launched"
        # "Exit - Exit the application."
        n271 = call "Application Name--constant.vi"() -> ("Application Name"=w524:string)  [unwired: 11 in]
        n272 = call "Stop Module.vi"("Wait for Module to Stop? (F)"=w523, "Origin"=w524) -> ("error out"=w534:errorcluster)  [unwired: 9 in]
        n273 = call "Stop Module.vi"("Wait for Module to Stop? (F)"=w523, "Origin"=w524) -> ("error out"=w529:errorcluster)  [unwired: 9 in]
        n274 = call "Stop Module.vi"("Wait for Module to Stop? (F)"=w523, "Origin"=w524) -> ("error out"=w528:errorcluster)  [unwired: 9 in]
        n275 = call "Stop Module.vi"("Wait for Module to stop? (F)"=w523, "Origin"=w524, "Module ID"=-1) -> ("error out"=w522:errorcluster)  [unwired: 8 in]
        n276 = Merge Errors(w522, w534, w529, w528) -> (w535:errorcluster)
      }
    }
    n277 = Or(x=w114, y=w110) -> (x .or. y?=w108:bool)
  }
  n278 = Unregister For Events(event registration refnum=w86) -> ()  [unwired: 1 in, 1 out]
  n279 = call <vilib>:"Simple Error Handler.vi"("error in (no error)"=w93) -> ("error out"=w92:errorcluster)  [unwired: 4 in, 4 out]
  n280 = disable-structure "Conditional Disable Structure" shown="RUN_TIME_ENGINE==True" {
    disable-tunnel: w92 -> [_ _]
    frame condition #0 (active) {
    }
    frame condition #1 {
      # "Call Quit LabVIEW if running as a built application."
      n281 = Quit LabVIEW(quit? (T)=TRUE) -> ()
    }
  }
